vi "EX 12-1Tracking.vi"() -> ()   [LabVIEW 2011]
uses:
  <vilib>/LabVIEW Interface for Arduino/Type Defs/Board Type.ctl
  <vilib>/LabVIEW Interface for Arduino/Type Defs/Connection Type.ctl
  <vilib>/LabVIEW Interface for Arduino/LabVIEW Interface for Arduino.lvlib
panel:
  out "Degrees Y":u8=100
  out "Center of Y":dbl=249.56985871271584
  out "Degrees X":u8=89
  in  "Number of Servos":u8=2
  out "Image Out":T1(plugin-control)
  in  "Stop (F)":bool
  out "Image Out 2":T1(plugin-control)
  out "Center of X":dbl=302.50104657247516
  out "Area":dbl=3822.0
  in  "Tab Control":enum32{"Vision Scale", "Tracking Gain"}(tab)
  in  "Selection Values":T2(array[cluster])=[{"Measurement Parameter"=35, "Range Lower Value"=1000.0, "Range Upper Value"=60000.0, "Range"=FALSE, "Measurement Type"=FALSE}] {"Measurement Parameter" items=["Center of Mass X", "Center of Mass Y", "First Pixel X", "First Pixel Y", "Bounding Rect Left", "Bounding Rect Top", "Bounding Rect Right", "Bounding Rect Bottom", "Max Feret Diameter Start X", "Max Feret Diameter Start Y", "Max Feret Diameter End X", "Max Feret Diameter End Y", "Max Horiz. Segment Length Left", "Max Horiz. Segment Length Right", "Max Horiz. Segment Length Row", "-", "Bounding Rect Width", "Bounding Rect Height", "Bounding Rect Diagonal", "Perimeter", "Convex Hull Perimeter", "Holes' Perimeter", "Max Feret Diameter", "Equivalent Ellipse Major Axis", "Equivalent Ellipse Minor Axis", "Equivalent Ellipse Minor Axis (Feret)", "Equivalent Rect Long Side", "Equivalent Rect Short Side", "Equivalent Rect Diagonal", "Equivalent Rect Short Side (Feret)", "Average Horiz. Segment Length", "Average Vert. Segment Length", "Hydraulic Radius", "Waddel Disk Diameter", "-", "Area", "Holes' Area", "Particle & Holes' Area", "Convex Hull Area", "Image Area", "-", "Number of Holes", "Number of Horiz. Segments", "Number of Vert. Segments", "-", "Orientation", "Max Feret Diameter Orientation", "-", "% Area/Image Area", "% Area/(Particle & Holes' Area)", "Ratio of Equivalent Ellipse Axes", "Ratio of Equivalent Rect Sides", "-", "Elongation Factor", "Compactness Factor", "Heywood Circularity Factor", "Type Factor", "-", "Sum X", "Sum Y", "Sum XX", "Sum XY", "Sum YY", "Sum XXX", "Sum XXY", "Sum XYY", "Sum YYY", "-", "Moment of Inertia XX", "Moment of Inertia XY", "Moment of Inertia YY", "Moment of Inertia XXX", "Moment of Inertia XXY", "Moment of Inertia XYY", "Moment of Inertia YYY", "Norm. Moment of Inertia XX", "Norm. Moment of Inertia XY", "Norm. Moment of Inertia YY", "Norm. Moment of Inertia XXX", "Norm. Moment of Inertia XXY", "Norm. Moment of Inertia XYY", "Norm. Moment of Inertia YYY", "Hu Moment 1", "Hu Moment 2", "Hu Moment 3", "Hu Moment 4", "Hu Moment 5", "Hu Moment 6", "Hu Moment 7"]}
  in  "Blue or Luma or Val or Inten Range":cluster{"Lower value":i32, "Upper value":i32}={"Lower value"=0, "Upper value"=80} {"Lower value" scale=0.0..255.0; "Upper value" scale=0.0..255.0}
  in  "Green or Sat Range":cluster{"Lower value":i32, "Upper value":i32}={"Lower value"=139, "Upper value"=255} {"Lower value" scale=0.0..255.0; "Upper value" scale=0.0..255.0}
  in  "Red or Hue Range":cluster{"Lower value":i32, "Upper value":i32}={"Lower value"=214, "Upper value"=255} {"Lower value" scale=0.0..255.0; "Upper value" scale=0.0..255.0}
  in  "Number of Erosion":i32=1
  in  "Color Mode":u16(ring)=1 items=["RGB", "HSL", "HSV", "HSI"]
  in  "Gain Y":dbl=0.3
  in  "Gain X":dbl=0.45
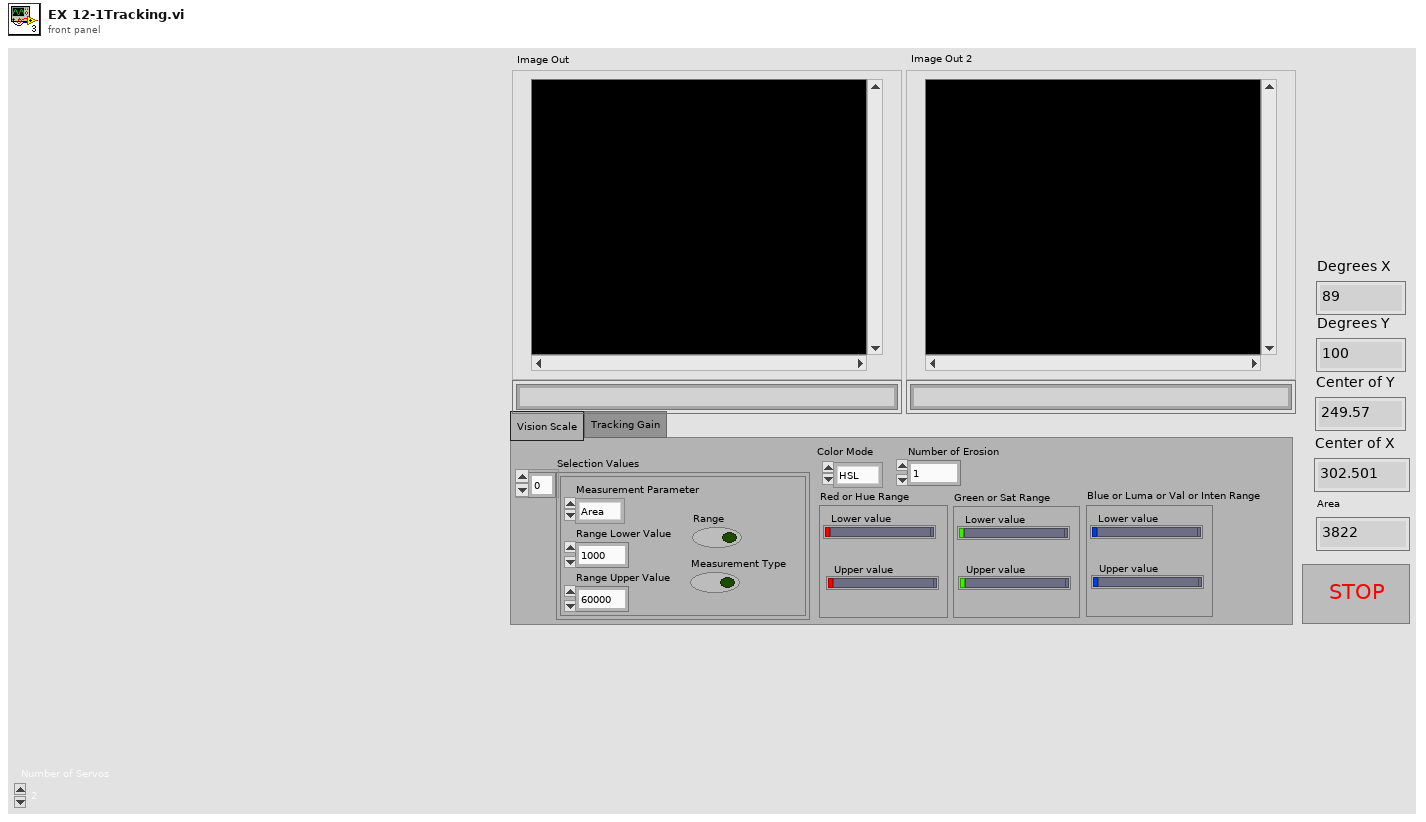
[diagram p1: front panel]
types:
  T1 = typedef "IMAQ Image.ctl" = refnum<image>
  T2 = cluster{"Measurement Parameter":i32, "Range Lower Value":dbl, "Range Upper Value":dbl, "Range":bool, "Measurement Type":bool}[]
  T3 = typedef "LabVIEW Interface for Arduino.lvlib/Connection Type.ctl" = enum8{"USB / Serial", "XBEE", "BlueSmirf (Bluetooth)"}
  T4 = typedef "LabVIEW Interface for Arduino.lvlib/Board Type.ctl" = enum16{"Uno", "Dimuelanove w/Atmega 328", "Mega 2560"}
  T5 = typedef "LabVIEW Interface for Arduino.lvlib/Arduino Resource.ctl" = cluster{"VISA resource":refnum<visa-resource-name>, "Board Type":T4, "Connection Type":enum8{"USB / Serial"}, "Bytes Per Packet (15)":u8}
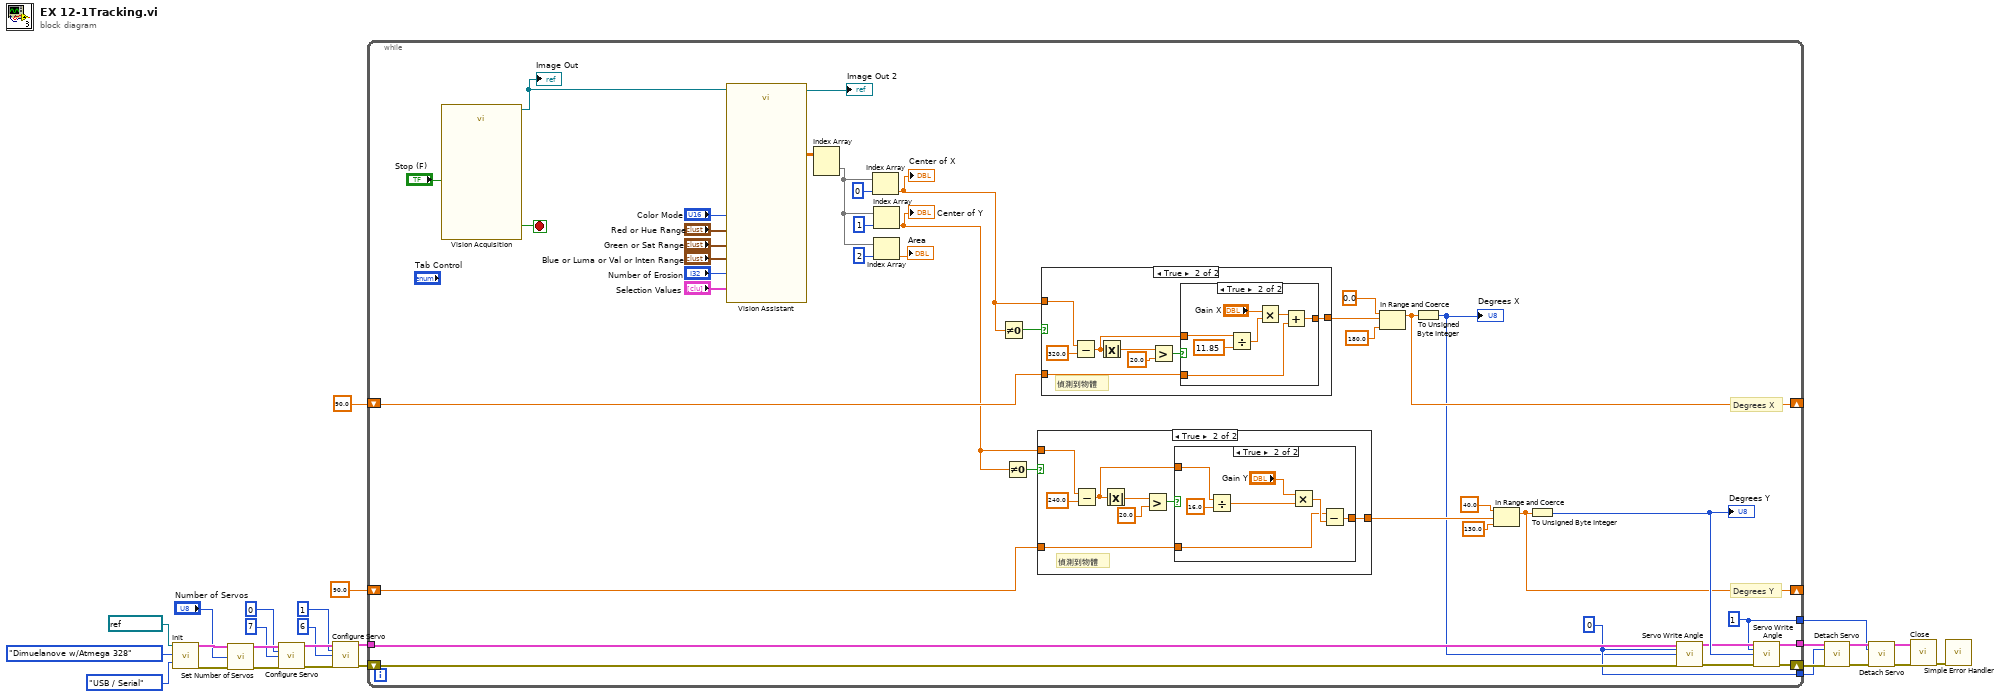
[diagram p0: block diagram]
diagram:
  n1 = call <vilib>:"Init.vi"("VISA resource"=refnum<visa-resource-name> "COM3", "Board Type (Uno)"=Board_Type."Dimuelanove w/Atmega 328", "Connection Type (USB/Serial)"=Connection_Type."USB / Serial") -> ("Arduino Resource"=w27:T5, "error out"=w26:errorcluster)  [unwired: 15 in]
  n2 = call <vilib>:"Set Number of Servos.vi"("Arduino Resource"=w27, "Number Of Servos (1)"="Number of Servos", "error in"=w26) -> ("Arduino Resource"=w24:T5, "error out"=w23:errorcluster)  [unwired: 11 in]
  n3 = call <vilib>:"Configure Servo.vi"("Arduino Resource"=w24, "Servo Number (0)"=u8 0 ("Servo Number"), "DIO Pin (2)"=u8 7 ("Servo Number"), "error in"=w23) -> ("Arduino Resource"=w22:T5, "error out"=w21:errorcluster)  [unwired: 10 in]
  n4 = call <vilib>:"Configure Servo.vi"("Arduino Resource"=w22, "Servo Number (0)"=u8 1 ("Servo Number"), "DIO Pin (2)"=u8 6 ("Servo Number"), "error in"=w21) -> ("Arduino Resource"=w12:T5, "error out"=w13:errorcluster)  [unwired: 10 in]
  n5 = while {
    shift-right: [w34] -> w8
    shift-left: w13 -> [w53]
    tunnel: w12 -> [w52]
    tunnel: [w35] -> w9
    shift-right: [w46] -> _
    shift-left: 90.0 -> [w29]
    tunnel: [w50] -> w7
    shift-right: [w31] -> _
    shift-left: 90.0 -> [w42]
    tunnel: [w32] -> w1
    stop <- w67 stop-if-true
    w50 = u8 0 ("Servo Number")
    w32 = u8 1 ("Servo Number")
    # "Degrees Y"
    # "Degrees X"
    n6 = call "Vision Acquisition"("Stop (F)"="Stop (F)") -> ("Image Out"=w66:T1, "Stopped"=w67:bool)  [unwired: 22 in, 3 out]
    "Image Out" <- w66
    n7 = call "Vision Assistant"("Image In"=w66, "Color Mode (Color Threshold 1)"="Color Mode", "Red or Hue Range (Color Threshold 1)"="Red or Hue Range", "Green or Sat Range (Color Threshold 1)"="Green or Sat Range", "Blue or Luma or Val or Inten Range (Color Threshold 1)"="Blue or Luma or Val or Inten Range", "Number of Erosion (Adv. Morphology 1)"="Number of Erosion", "Selection Values (Particle Filter 1)"="Selection Values") -> ("Image Out"=→"Image Out 2":T1, "Particle Measurements (Pixels) (Particle Analysis 1)"=w63:dbl[][])  [unwired: 17 in, 2 out]
    n8 = Index Array(array=w63) -> (element=w30:dbl[])  [unwired: 2 in]
    n9 = Index Array(array=w30, index=0) -> (element=w37:dbl)
    "Center of X" <- w37
    n10 = Index Array(array=w30, index=1) -> (element=w28:dbl)
    "Center of Y" <- w28
    n11 = Index Array(array=w30, index=2) -> (element=→"Area":dbl)
    n12 = Not Equal To 0?(x=w37) -> (x != 0?=w51:bool)
    n13 = Not Equal To 0?(x=w28) -> (x != 0?=w43:bool)
    n14 = case shown="True" w43 {
      tunnel: [w68 w70] -> w39
      tunnel: w42 -> [w68 w71]
      tunnel: w28 -> [_ w69]
      frame False {
        # "未偵測到物體"
        # "If no object, Center = 0."
      }
      frame True {
        # "偵測到物體"
        n15 = Subtract(x=w69, y=240.0) -> (x-y=w72:dbl)
        n16 = Absolute Value(x=w72) -> (abs(x)=w75:dbl)
        n17 = Greater?(x=w75, y=20.0) -> (0:w73:bool)
        n18 = case shown="True" w73 {
          tunnel: w71 -> [w77 w78]
          tunnel: [w77 w83] -> w70
          tunnel: w72 -> [_ w82]
          frame False {
          }
          frame True {
            n19 = Divide(x=w82, y=16.0) -> (x/y=w79:dbl)
            n20 = Multiply(x="Gain Y", y=w79) -> (x*y=w81:dbl)
            n21 = Subtract(x=w78, y=w81) -> (x-y=w83:dbl)
          }
        }
      }
    }
    n22 = case shown="True" w51 {
      tunnel: w37 -> [_ w89]
      tunnel: [w85 w86] -> w49
      tunnel: w29 -> [w85 w87]
      frame False {
        # "未偵測到物體"
      }
      frame True {
        # "偵測到物體"
        n23 = Subtract(x=w89, y=320.0) -> (x-y=w88:dbl)
        n24 = Absolute Value(x=w88) -> (abs(x)=w92:dbl)
        n25 = Greater?(x=w92, y=20.0) -> (0:w90:bool)
        n26 = case shown="True" w90 {
          tunnel: w88 -> [_ w100]
          tunnel: w87 -> [w94 w99]
          tunnel: [w94 w98] -> w86
          frame False {
          }
          frame True {
            n27 = Divide(x=w100, y=11.85) -> (x/y=w96:dbl)
            n28 = Multiply(x="Gain X", y=w96) -> (x*y=w97:dbl)
            n29 = Add(x=w97, y=w99) -> (x+y=w98:dbl)
          }
        }
      }
    }
    n30 = In Range and Coerce(upper limit=0.0, x=w49, lower limit=180.0) -> (coerced(x)=w46:dbl)  [unwired: 1 out]
    n31 = To Unsigned Byte Integer(number=w46) -> (unsigned 8bit integer=w38:u8)
    "Degrees X" <- w38
    n32 = In Range and Coerce(upper limit=40.0, x=w39, lower limit=130.0) -> (coerced(x)=w31:dbl)  [unwired: 1 out]
    n33 = To Unsigned Byte Integer(number=w31) -> (unsigned 8bit integer=w44:u8)
    "Degrees Y" <- w44
    n34 = call <vilib>:"Servo Write Angle.vi"("Arduino Resource"=w52, "Servo Number"=w50, "Angle (Degrees)"=w38, "error in"=w53) -> ("Arduino Resource"=w36:T5, "error out"=w33:errorcluster)  [unwired: 10 in]
    n35 = call <vilib>:"Servo Write Angle.vi"("Arduino Resource"=w36, "Servo Number"=w32, "Angle (Degrees)"=w44, "error in"=w33) -> ("Arduino Resource"=w35:T5, "error out"=w34:errorcluster)  [unwired: 10 in]
  }
  n36 = call <vilib>:"Detach Servo.vi"("Arduino Resource"=w9, "Servo Number"=w7, "error in"=w8) -> ("Arduino Resource"=w5:T5, "error out"=w3:errorcluster)  [unwired: 11 in]
  n37 = call <vilib>:"Detach Servo.vi"("Arduino Resource"=w5, "Servo Number"=w1, "error in"=w3) -> ("Arduino Resource"=w4:T5, "error out"=w2:errorcluster)  [unwired: 11 in]
  n38 = call <vilib>:"Close.vi"("Arduino Resource"=w4, "error in"=w2) -> ("error out"=w11:errorcluster)  [unwired: 13 in]
  n39 = call <vilib>:"Simple Error Handler.vi"("error in (no error)"=w11) -> ()  [unwired: 4 in, 5 out]
